vi "Do.vi"(8 "error in":errorcluster, 10 "Actor in":refnum<class "Actor.lvclass">, 11 "Stop PAS Wvfm Write MSG":refnum<class "Stop PAS Wvfm Write MSG.lvclass">) -> (0 "error out":errorcluster, 2 "Actor out":refnum<class "Actor.lvclass">)   [LabVIEW 2014, in "Controller.lvlib" / "Stop PAS Wvfm Write MSG.lvclass"]
doc: "(<B>Filename</B>: Actor Framework.lvlib:Message.lvclass:Do.vi)\n\nDefines what a message does when it is received by an actor. Generally, a message instructs an actor to invoke one of its methods. By default, this method does nothing. A child class must override it to define behavior. Create a child class by using the Actor Framework Message Maker dialog box."
uses:
  Stop PAS Wvfm Write MSG.lvclass
  <vilib>/ActorFramework/Actor/Actor.lvclass
  Controller.lvclass
  Controller.lvclass/Controller.ctl
  Controls/eMap.ctl
  <vilib>/ActorFramework/Message Enqueuer/Message Enqueuer.lvclass
  <vilib>/ActorFramework/Message Enqueuer/Message Enqueuer.lvclass/Message Enqueuer.ctl
  Accessors/Read Enqueuer Map.vi
  Accessors/Write Enqueuer Map.vi
  <vilib>/ActorFramework/Message Enqueuer/Enqueue.vi
  <vilib>/ActorFramework/Message Priority Queue/Priority Enqueue.vi
  <vilib>/ActorFramework/Stop Msg/Stop Msg.lvclass
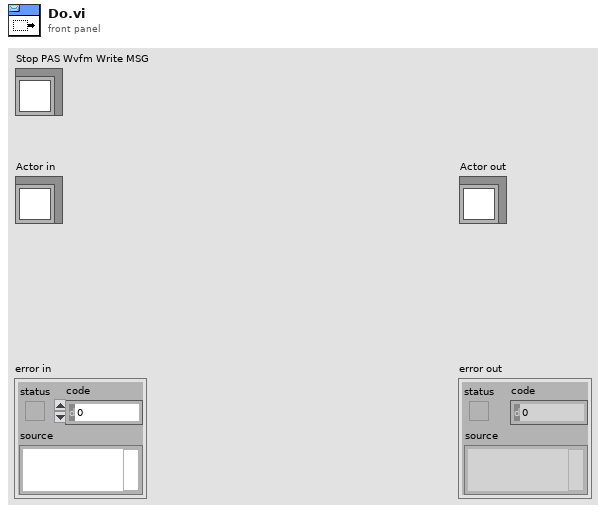
[diagram p1: front panel]
types:
  T1 = typedef "Controller.lvlib/Controller.lvclass/eMap.ctl" = cluster{"Enqueuer":refnum<class "Message Enqueuer.lvclass">, "Active":bool}
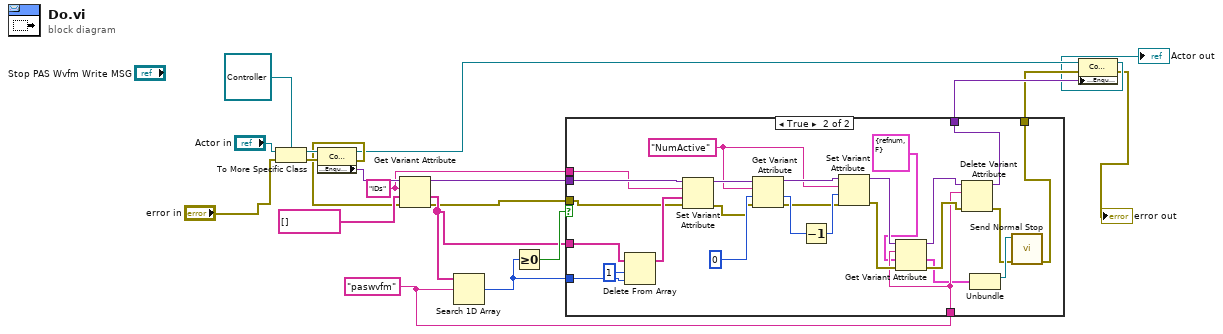
[diagram p0: block diagram]
diagram:
  w6 = "paswvfm" ("element")
  w9 = "IDs" ("name")
  n1 = To More Specific Class(target class=refnum<class "Controller.lvclass"> refnum ("Controller:Controller"), reference="Actor in", error in="error in") -> (specific class reference=w17:refnum<class "Controller.lvclass">, error out=w16:errorcluster)
  n2 = property class="Controller"(reference=w17, error in=w16) -> (reference out=w5:refnum<class "Controller.lvclass">, error out=w7:errorcluster, "Accessors:Enqueuer Map"=w15:variant)
  n3 = Get Variant Attribute(Variant=w15, name=w9, default value (empty Variant)=string[] [], error in=w7) -> (duplicate Variant=w13:variant, value=w10:string[], error out=w8:errorcluster)  [unwired: 1 out]
  n4 = Search 1D Array(1D array=w10, element=w6) -> (index of element=w11:i32)  [unwired: 1 in]
  n5 = Greater Or Equal To 0?(x=w11) -> (x >= 0?=w12:bool)
  n6 = case shown="True" w12 {
    tunnel: w13 -> [w21 w48]
    tunnel: w11 -> [_ w47]
    tunnel: w10 -> [_ w45]
    tunnel: w9 -> [_ w43]
    tunnel: w8 -> [w22 w34]
    tunnel: w6 -> [_ w28]
    tunnel: [w21 w33] -> w4
    tunnel: [w22 w23] -> w3
    frame False {
    }
    frame True {
      w37 = "NumActive" ("name")
      n7 = Delete From Array(array=w45, length=1, index=w47) -> (array with subset deleted=w44:string[])  [unwired: 1 out]
      n8 = Set Variant Attribute(Variant=w48, name=w43, value=w44, error in=w34) -> (Variant out=w42:variant, error out=w35:errorcluster)  [unwired: 1 out]
      n9 = Get Variant Attribute(Variant=w42, name=w37, default value (empty Variant)=i16 0, error in=w35) -> (duplicate Variant=w38:variant, value=w40:i16, error out=w36:errorcluster)  [unwired: 1 out]
      n10 = Decrement(x=w40) -> (x-1=w39:i16)
      n11 = Set Variant Attribute(Variant=w38, name=w37, value=w39, error in=w36) -> (Variant out=w32:variant, error out=w29:errorcluster)  [unwired: 1 out]
      n12 = Get Variant Attribute(Variant=w32, name=w28, default value (empty Variant)=T1 {"Enqueuer"=refnum, "Active"=FALSE} ("eMap"), error in=w29) -> (duplicate Variant=w31:variant, value=w26:T1, error out=w30:errorcluster)  [unwired: 1 out]
      n13 = Delete Variant Attribute(4:w30, 6:w28, 7:w31) -> (0:w24:errorcluster, 3:w33:variant)  [unwired: 1 out]
      n14 = Unbundle(w26) -> ("Enqueuer"=w25:refnum<class "Message Enqueuer.lvclass">)  [unwired: 1 out]
      n15 = call <vilib>:"Send Normal Stop.vi"("error in (no error)"=w24, "Message Enqueuer"=w25) -> ("error out"=w23:errorcluster)  [unwired: 9 in]
    }
  }
  n16 = property class="Controller"(reference=w5, error in=w3, "Accessors:Enqueuer Map"=w4) -> (reference out=→"Actor out":refnum<class "Controller.lvclass">, error out=→"error out":errorcluster)
